vi "StreamBus.Do.vi"(10 "State Variables":T2, 11 "gRPCid":T1) -> (2 "State Variables out":T2)   [LabVIEW 2025, in "bus_monitor_server_do.lvlib"]
uses:
  bus_monitor_server_do.lvlib
  SubVIs/StreamProcess.Main.vi
  <vilib>/gRPC/LabVIEW gRPC Library/Shared/grpcId.ctl
  <vilib>/gRPC/LabVIEW gRPC Library/grpc-lvsupport-release.lvlib
  Types/StreamProcess.InputRefs.ctl
  Types/StreamProcess.VIRef.ctl
  bus_monitor_server/RPC Messages/ni_bus_monitor_api_Frame.ctl
  bus_monitor_server/bus_monitor_server.lvlib
  bus_monitor_server/RPC Messages/ni_bus_monitor_api_StreamBusReply.ctl
  bus_monitor_server/RPC Service/Bus_Monitor_API/Bus_Monitor_API.lvclass
  bus_monitor_server/RPC Messages/ni_bus_monitor_api_ErrorInfo.ctl
  bus_monitor_server/RPC Messages/ni_bus_monitor_api_LastCommError.ctl
  bus_monitor_server/RPC Messages/ni_bus_monitor_api_CommState.ctl
  bus_monitor_server/RPC Messages/ni_bus_monitor_api_CanCommState.ctl
  bus_monitor_server/RPC Messages/ni_bus_monitor_api_FrameFilter.ctl
  bus_monitor_server/RPC Messages/ni_bus_monitor_api_DirectionFilter.ctl
  bus_monitor_server/RPC Messages/ni_bus_monitor_api_FilterInfo.ctl
  Types/XNET.InitialSettings.ctl
  Types/StreamProcess.Refs.ctl
  Types/MainProcess.StateVariables.ctl
  bus_monitor_server/RPC Messages/ni_bus_monitor_api_FdIsoMode.ctl
  bus_monitor_server/RPC Messages/ni_bus_monitor_api_Termination.ctl
  bus_monitor_server/RPC Messages/ni_bus_monitor_api_CanMode.ctl
  bus_monitor_server/RPC Messages/ni_bus_monitor_api_ConnectSettings.ctl
  bus_monitor_server/RPC Messages/ni_bus_monitor_api_Session.ctl
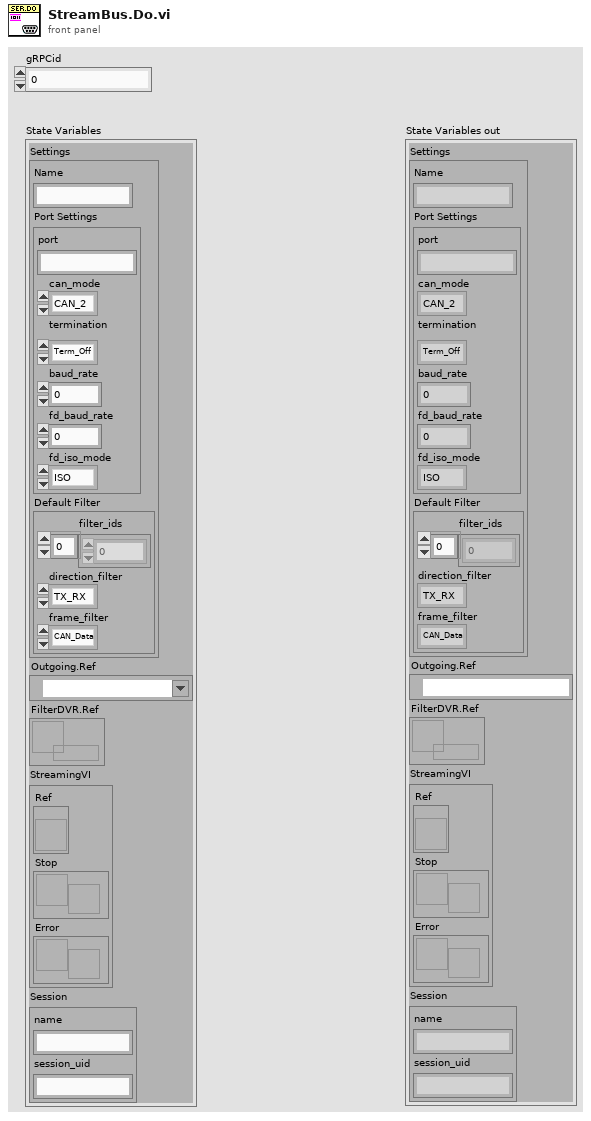
[diagram p1: front panel]
types:
  T1 = typedef "grpc-lvsupport-release.lvlib/grpcId.ctl" = u64
  T2 = typedef "bus_monitor_server_do.lvlib/MainProcess.StateVariables.ctl" = cluster{"Settings":T3, "Outgoing.Ref":refnum<k21>, "FilterDVR.Ref":refnum<data-value>, "StreamingVI":T11, "Session":T13}
  T3 = typedef "bus_monitor_server_do.lvlib/XNET.InitialSettings.ctl" = cluster{"Name":string, "Port Settings":T4, "Default Filter":T8}
  T4 = typedef "bus_monitor_server.lvlib/ni_bus_monitor_api_ConnectSettings.ctl" = cluster{"port":string, "can_mode":T5, "termination":T6, "baud_rate":u64, "fd_baud_rate":u64, "fd_iso_mode":T7}
  T5 = typedef "bus_monitor_server.lvlib/ni_bus_monitor_api_CanMode.ctl" = enum32{"CAN_2", "CAN_FD", "CAN_FD_BRS"}
  T6 = typedef "bus_monitor_server.lvlib/ni_bus_monitor_api_Termination.ctl" = enum32{"Term_Off", "Term_On"}
  T7 = typedef "bus_monitor_server.lvlib/ni_bus_monitor_api_FdIsoMode.ctl" = enum32{"ISO", "Non_ISO", "ISO_Legacy"}
  T8 = typedef "bus_monitor_server.lvlib/ni_bus_monitor_api_FilterInfo.ctl" = cluster{"filter_ids":u32[], "direction_filter":T9, "frame_filter":T10}
  T9 = typedef "bus_monitor_server.lvlib/ni_bus_monitor_api_DirectionFilter.ctl" = enum32{"TX_RX", "RX", "TX"}
  T10 = typedef "bus_monitor_server.lvlib/ni_bus_monitor_api_FrameFilter.ctl" = enum32{"CAN_Data", "CAN_Remote", "CAN_Bus_Error", "CAN_2_Data", "CAN_FD_Data", "CAN_FD_BRS_Data", "J1939_Data", "Delay", "Log_Trigger", "Start_Trigger", "All"}
  T11 = typedef "bus_monitor_server_do.lvlib/StreamProcess.Refs.ctl" = cluster{"Ref":T12, "Stop":refnum<notifier>, "Error":refnum<notifier>}
  T12 = typedef "bus_monitor_server_do.lvlib/StreamProcess.VIRef.ctl" = refnum<vi>
  T13 = typedef "bus_monitor_server.lvlib/ni_bus_monitor_api_Session.ctl" = cluster{"name":string, "session_uid":string}
  T14 = typedef "bus_monitor_server.lvlib/ni_bus_monitor_api_StreamBusRequest.ctl" = cluster{"session":T13}
  T15 = typedef "bus_monitor_server.lvlib/ni_bus_monitor_api_StreamBusReply.ctl" = cluster{"can_comm_state":T16, "frame":T19[], "error":T20}
  T16 = typedef "bus_monitor_server.lvlib/ni_bus_monitor_api_CanCommState.ctl" = cluster{"fault_code":i32, "fault":bool, "comm_state":T17, "last_comm_error":T18, "receive_error_counter":u32, "transmit_error_counter":u32, "transceiver_error":bool, "sleep":bool}
  T17 = typedef "bus_monitor_server.lvlib/ni_bus_monitor_api_CommState.ctl" = enum32{"Error_Active", "Error_Passive", "Bus_Off", "Init"}
  T18 = typedef "bus_monitor_server.lvlib/ni_bus_monitor_api_LastCommError.ctl" = enum32{"None", "Stuff", "Form", "ACK", "Bit1", "Bit0", "CRC"}
  T19 = typedef "bus_monitor_server.lvlib/ni_bus_monitor_api_Frame.ctl" = cluster{"timestamp":dbl, "payload":u8[], "identifier":u32, "frame_type":u32, "extended":bool, "echo":bool}
  T20 = typedef "bus_monitor_server.lvlib/ni_bus_monitor_api_ErrorInfo.ctl" = errorcluster
  T21 = typedef "bus_monitor_server_do.lvlib/StreamProcess.InputRefs.ctl" = cluster{"ReportError":refnum<notifier>, "CheckStop":refnum<notifier>, "gRPCid":T1}
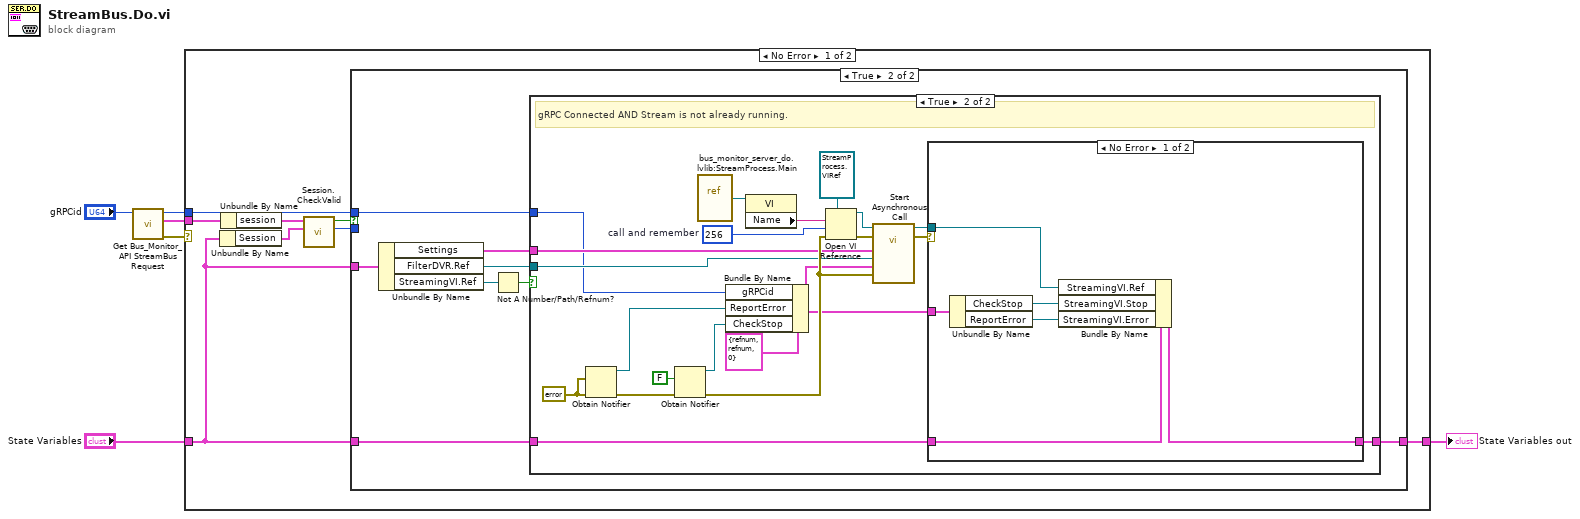
[diagram p0: block diagram]
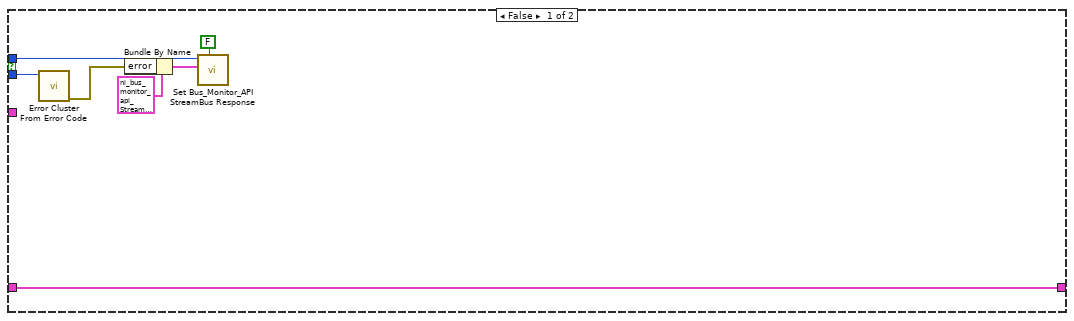
[diagram p2: hidden frame]
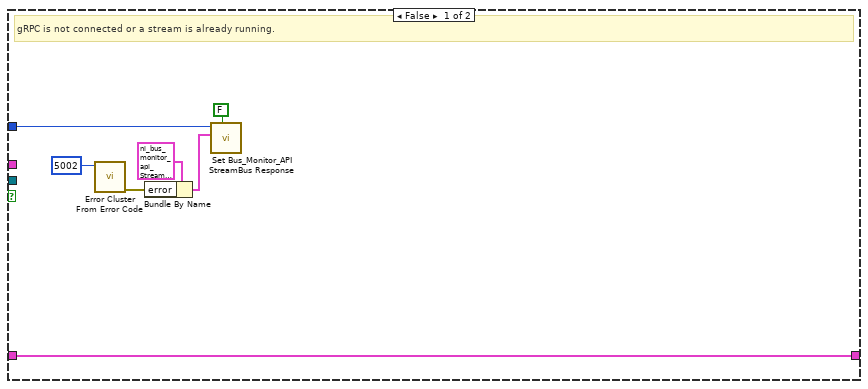
[diagram p3: hidden frame]
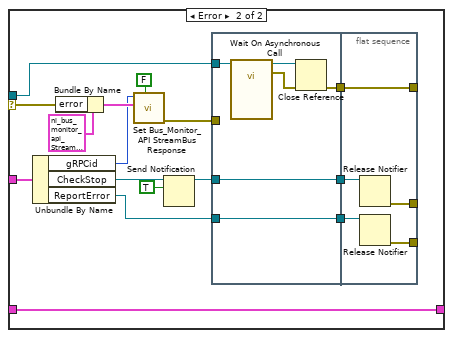
[diagram p4: hidden frame]
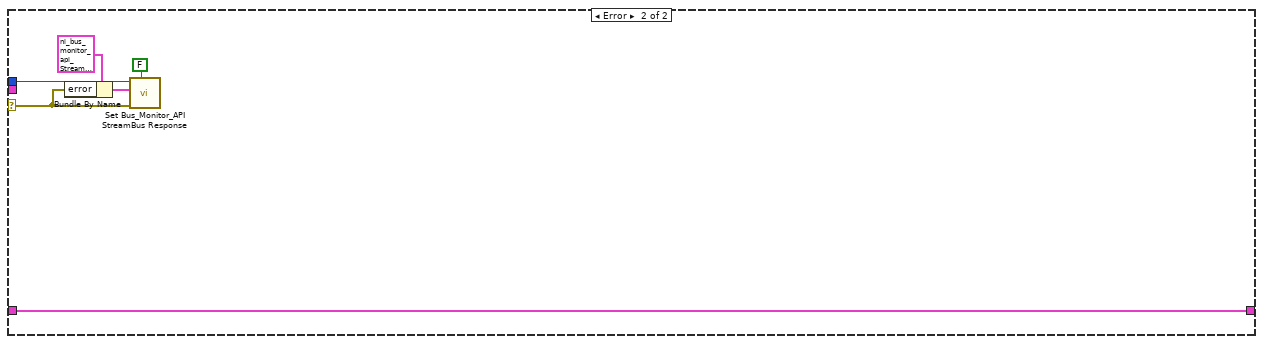
[diagram p5: hidden frame]
diagram:
  n1 = call "Get Bus_Monitor_API StreamBus Request.vi"("gRPCid"="gRPCid") -> ("error out"=w2:errorcluster, "Message Data"=w1:T14, "gRPCid out"=w3:T1)  [unwired: 8 in]
  n2 = case shown="No Error" w2 {
    selector: w2 -> [_ w90]
    tunnel: "State Variables" -> [w7 w91]
    tunnel: [w14 w91] -> w5
    tunnel: w3 -> [w13 w92]
    tunnel: w1 -> [w12 _]
    frame No Error {
      n3 = Unbundle By Name(w7) -> ("Session"=w10:T13)
      n4 = Unbundle By Name(w12) -> ("session"=w11:T13)
      n5 = call "Session.CheckValid.vi"("Cached Session"=w10, "requested session"=w11) -> ("Error Code"=w8:i32, "Valid?"=w9:bool)  [unwired: 8 in]
      n6 = case shown="True" w9 {
        tunnel: [w15 w26] -> w14
        tunnel: w13 -> [w18 w24]
        tunnel: w7 -> [_ w23]
        tunnel: w8 -> [w17 _]
        tunnel: w7 -> [w15 _]
        frame False {
          n7 = call <vilib>:"Error Cluster From Error Code.vi"("error code (0)"=w17) -> ("error out"=w16:errorcluster)  [unwired: 8 in]
          n8 = Bundle By Name(cluster=T15 {"can_comm_state"={"fault_code"=0, "fault"=FALSE, "comm_state"=enum."Error_Active", "last_comm_error"=enum."None", "receive_error_counter"=0, "transmit_error_counter"=0, "transceiver_error"=FALSE, "sleep"=FALSE}, "frame"=[], "error"={"status"=FALSE, "code"=0, "source"=""}} ("Message Data"), "error"=w16) -> (w19:T15)
          n9 = call "Set Bus_Monitor_API StreamBus Response.vi"("Streaming? (F)"=FALSE, "Message Data"=w19, "gRPCid in"=w18) -> ()  [unwired: 8 in, 1 out]
        }
        frame True {
          n10 = Unbundle By Name(w23) -> ("Settings"=w27:T3, "FilterDVR.Ref"=w28:refnum<data-value>, "StreamingVI.Ref"=w25:T12)
          n11 = Not A Number/Path/Refnum?(number/path/refnum=w25) -> (NaN/Path/Refnum?=w22:bool)
          n12 = case shown="True" w22 {
            tunnel: w24 -> [w30 w37]
            tunnel: w27 -> [_ w45]
            tunnel: w28 -> [_ w44]
            tunnel: w23 -> [w31 w43]
            tunnel: [w31 w42] -> w26
            frame False {
              # "gRPC is not connected or a stream is already running."
              n13 = call <vilib>:"Error Cluster From Error Code.vi"("error code (0)"=5002) -> ("error out"=w32:errorcluster)  [unwired: 8 in]
              n14 = Bundle By Name(cluster=T15 {"can_comm_state"={"fault_code"=0, "fault"=FALSE, "comm_state"=enum."Error_Active", "last_comm_error"=enum."None", "receive_error_counter"=0, "transmit_error_counter"=0, "transceiver_error"=FALSE, "sleep"=FALSE}, "frame"=[], "error"={"status"=FALSE, "code"=0, "source"=""}} ("Message Data"), "error"=w32) -> (w33:T15)
              n15 = call "Set Bus_Monitor_API StreamBus Response.vi"("Streaming? (F)"=FALSE, "Message Data"=w33, "gRPCid in"=w30) -> ()  [unwired: 8 in, 1 out]
            }
            frame True {
              w49 = errorcluster {"status"=FALSE, "code"=0, "source"=""} ("error in (no error)")
              w55 = 256  # call and remember
              # "gRPC Connected AND Stream is not already running."
              n16 = Obtain Notifier(notification data type=w49, error in (no error)=w49) -> (notifier out=w39:refnum<notifier>, error out=w52:errorcluster)  [unwired: 2 in, 1 out]
              n17 = Obtain Notifier(notification data type=FALSE, error in (no error)=w52) -> (notifier out=w40:refnum<notifier>, error out=w47:errorcluster)  [unwired: 2 in, 1 out]
              n18 = vi-ref "bus_monitor_server_do.lvlib:StreamProcess.Main.vi"() -> (w48:refnum<vi>)
              n19 = Bundle By Name(cluster=T21 {"ReportError"=refnum, "CheckStop"=refnum, "gRPCid"=0}, "gRPCid"=w37, "ReportError"=w39, "CheckStop"=w40) -> (w36:T21)
              n20 = property class="VI"(reference=w48) -> ("Name"=w53:string)  [unwired: 1 in, 2 out]
              n21 = Open VI Reference(type specifier VI Refnum (for type only)=T12 refnum, vi path=w53, options=w55, error in (no error)=w47) -> (vi reference=w54:T12, error out=w56:errorcluster)  [unwired: 2 in]
              n22 = call-by-ref "Start Asynchronous Call"(reference=w54, error in=w56, 8:"error in (no error)"=w47, "Refs"=w36, "FilterDVR.Ref"=w44, "Settings"=w45) -> (reference out=w41:T12, error out=w38:errorcluster)  [unwired: 7 in, 1 out]
              n23 = case shown="No Error" w38 {
                selector: w38 -> [_ w68]
                tunnel: w43 -> [w62 w75]
                tunnel: [w61 w75] -> w42
                tunnel: w41 -> [w60 w76]
                tunnel: w36 -> [w59 w67]
                frame No Error {
                  n24 = Unbundle By Name(w59) -> ("CheckStop"=w58:refnum<notifier>, "ReportError"=w57:refnum<notifier>)
                  n25 = Bundle By Name(cluster=w62, "StreamingVI.Ref"=w60, "StreamingVI.Stop"=w58, "StreamingVI.Error"=w57) -> (w61:T2)
                }
                frame Error {
                  n26 = Unbundle By Name(w67) -> ("gRPCid"=w64:T1, "CheckStop"=w65:refnum<notifier>, "ReportError"=w66:refnum<notifier>)
                  n27 = Bundle By Name(cluster=T15 {"can_comm_state"={"fault_code"=0, "fault"=FALSE, "comm_state"=enum."Error_Active", "last_comm_error"=enum."None", "receive_error_counter"=0, "transmit_error_counter"=0, "transceiver_error"=FALSE, "sleep"=FALSE}, "frame"=[], "error"={"status"=FALSE, "code"=0, "source"=""}} ("Message Data"), "error"=w68) -> (w71:T15)
                  n28 = call "Set Bus_Monitor_API StreamBus Response.vi"("Streaming? (F)"=FALSE, "Message Data"=w71, "gRPCid in"=w64) -> ("error out"=w63:errorcluster)  [unwired: 8 in]
                  n29 = Send Notification(notification=TRUE, notifier=w65) -> (notifier out=w78:refnum<notifier>)  [unwired: 1 in, 1 out]
                  n30 = flat-sequence {
                    tunnel: w76 -> [w84]
                    tunnel: w78 -> [w80]
                    tunnel: w66 -> [w79]
                    tunnel: [w81] -> w74
                    tunnel: [w80] -> w73
                    tunnel: [w79] -> w72
                    tunnel: w63 -> [_]
                    tunnel: [w89] -> _
                    tunnel: w74 -> [w89]
                    tunnel: w73 -> [w88]
                    tunnel: w72 -> [w86]
                    tunnel: [w87] -> _
                    tunnel: [w85] -> _
                    frame #0 {
                      n31 = call-by-ref "Wait On Asynchronous Call"(reference=w84) -> (reference out=w83:T12, error out=w82:errorcluster)  [unwired: 12 in, 1 out]
                      n32 = Close Reference(reference=w83, error in (no error)=w82) -> (error out=w81:errorcluster)
                    }
                    frame #1 {
                      n33 = Release Notifier(notifier=w88) -> (error out=w87:errorcluster)  [unwired: 2 in, 2 out]
                      n34 = Release Notifier(notifier=w86) -> (error out=w85:errorcluster)  [unwired: 2 in, 2 out]
                    }
                  }
                }
              }
            }
          }
        }
      }
    }
    frame Error {
      n35 = Bundle By Name(cluster=T15 {"can_comm_state"={"fault_code"=0, "fault"=FALSE, "comm_state"=enum."Error_Active", "last_comm_error"=enum."None", "receive_error_counter"=0, "transmit_error_counter"=0, "transceiver_error"=FALSE, "sleep"=FALSE}, "frame"=[], "error"={"status"=FALSE, "code"=0, "source"=""}} ("Message Data"), "error"=w90) -> (w93:T15)
      n36 = call "Set Bus_Monitor_API StreamBus Response.vi"("Streaming? (F)"=FALSE, "error in (no error)"=w90, "Message Data"=w93, "gRPCid in"=w92) -> ()  [unwired: 7 in, 1 out]
    }
  }
  "State Variables out" <- w5
